vi "Update Label.vi"(8 "error in (no error)":errorcluster, 11 "Test Actor in":refnum<class "Example Actor.lvclass">) -> (0 "error out":errorcluster, 3 "Test Actor out":refnum<class "Example Actor.lvclass">)   [LabVIEW 2020, in "Example Actor.lvlib" / "Example Actor.lvclass"]
uses:
  Example Actor.lvclass
  C:/Program Files/National Instruments/LabVIEW 2020/vi.lib/MGI/Monitored Actor/Monitored Actor/Monitored Actor/Monitored Actor.lvclass
  <vilib>/MGI/Monitored Actor/Monitored Actor/Monitored Actor/Monitored Actor.lvclass
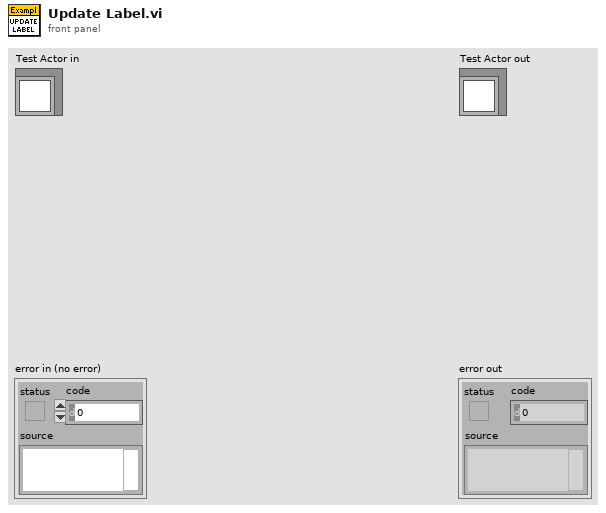
[diagram p1: front panel]
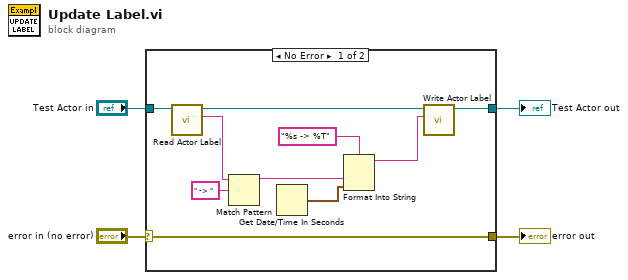
[diagram p0: block diagram]
diagram:
  n1 = case shown="No Error" "error in (no error)" {
    selector: "error in (no error)" -> [w14 w16]
    tunnel: [w14 w16] -> w3
    tunnel: [w6 w15] -> w1
    tunnel: "Test Actor in" -> [w13 w15]
    frame No Error {
      n2 = call <vilib>:"Read Actor Label.vi"("Monitored Actor in"=w13) -> ("Actor Label"=w8:string, "Monitored Actor out"=w12:refnum<class "Example Actor.lvclass">)  [unwired: 8 in, 1 out]
      n3 = Match Pattern(string=w8, regular expression=" -> ") -> (before substring=w9:string)  [unwired: 1 in, 3 out]
      n4 = Get Date/Time In Seconds() -> (seconds since 1Jan1904=w10:timestamp)
      n5 = Format Into String(format string="%s -> %T", w9, w10) -> (resulting string=w5:string)  [unwired: 2 in, 1 out]
      n6 = call-dynamic "Write Actor Label.vi"("Actor Label"=w5, "Monitored Actor in"=w12) -> ("Monitored Actor out"=w6:refnum<class "Example Actor.lvclass">)  [unwired: 8 in, 1 out]
    }
    frame Error {
    }
  }
  "error out" <- w3
  "Test Actor out" <- w1
